vi "Visa_Write read_UI GETPIN.vi"(0 "Simulado in":refnum<class "Simulado.lvclass">, 1 "VISA resource name":refnum<visa-resource-name>, 2 "Command to Send":string, 3 "Expected Response":string, 4 "Buttons":bool[](array[boolean]), 5 "error in (no error)":errorcluster) -> (13 "Valor pin":bool, 14 "Simulado out":refnum<class "Simulado.lvclass">, 15 "VISA resource name":refnum<visa-resource-name>, 16 "Response":string, 17 "Port":string, 18 "PIN":string, 19 "error out":errorcluster)   [LabVIEW 2020, in "Simulado.lvclass"]
uses:
  Simulado.lvclass
  UI Actor/UI Actor.lvclass
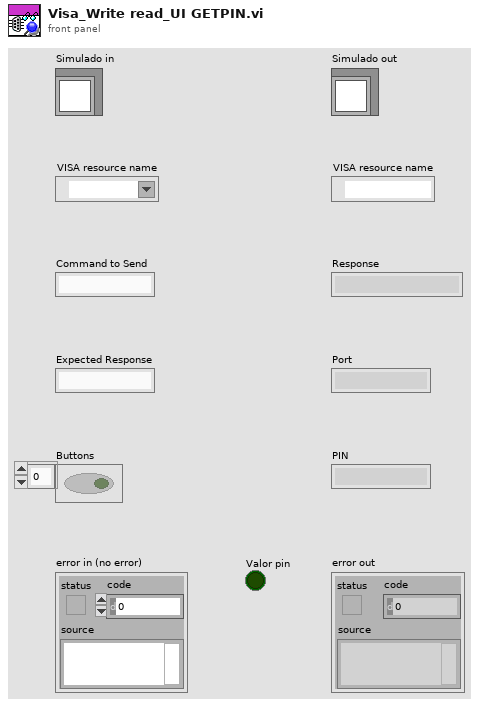
[diagram p1: front panel]
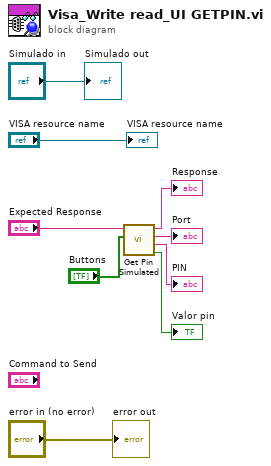
[diagram p0: block diagram]
diagram:
  n1 = call "Get Pin Simulated.vi"("Buttons"="Buttons", "Exprected Response"="Expected Response") -> ("Valor pin"=→"Valor pin":bool, "PIN"=→"PIN":string, "Port"=→"Port":string, "Response"=→"Response":string)  [unwired: 6 in]
  "error out" <- "error in (no error)"
  "Simulado out" <- "Simulado in"
  "VISA resource name" <- "VISA resource name"
